vi "ReadAutoPIDStart.vi"(8 "error in (no error)":errorcluster, 10 "Port Number":u16=2000, 11 "IP Address":string="192.168.12.200") -> (0 "error out":errorcluster, 2 "Output Diagnosis":dbl format="%.2f", 3 "PID Start":bool)   [LabVIEW 2013, in "ovenCtrl.lvlib"]
uses:
  ovenCtrl.lvlib
panel:
  # "Inputs"
  # "Outputs"
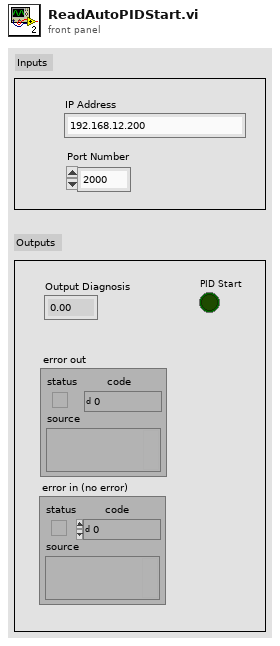
[diagram p1: front panel]
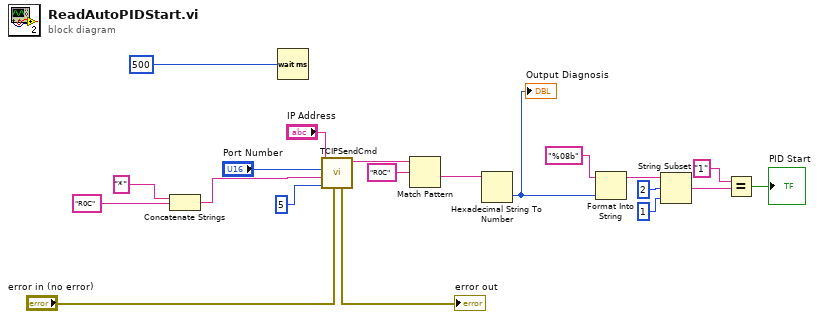
[diagram p0: block diagram]
diagram:
  n1 = Concatenate Strings("*" ("string"), "R0C" ("string")) -> (w15:string)
  n2 = Wait (ms)(milliseconds to wait=u32 500) -> ()  [unwired: 1 out]
  n3 = call "TCIPSendCmd.vi"("error in (no error)"="error in (no error)", "bytes to read"=5, "Command"=w15, "Port Number"="Port Number", "IP Address"="IP Address") -> ("Output Reading"=w10:string, "error out"=→"error out":errorcluster)  [unwired: 5 in]
  n4 = Match Pattern(string=w10, regular expression="R0C") -> (after substring=w9:string)  [unwired: 1 in, 3 out]
  n5 = Hexadecimal String To Number(string=w9) -> (number=w7:u32)  [unwired: 2 in, 1 out]
  "Output Diagnosis" <- w7
  n6 = Format Into String(format string="%08b", w7) -> (resulting string=w4:string)  [unwired: 2 in, 1 out]
  n7 = String Subset(string=w4, offset (0)=2, length (rest)=1 ("length (rest)")) -> (substring=w3:string)
  n8 = Equal?(x="1", y=w3) -> (x = y?=→"PID Start":bool)
